vi "ChangePWMDutyCycle.vi"(4 "Duty cycle (%)":dbl=50.0, 5 "Channel":i32, 6 "error in":errorcluster) -> (0 "error out":errorcluster)   [LabVIEW 2014]
doc: "Change the duty cycle of the PWM waveform.\n\nThe channel must be configured for PWM before calling this VI."
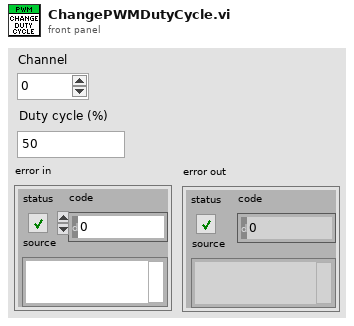
[diagram p1: front panel]
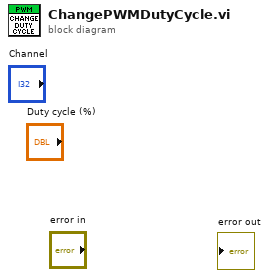
[diagram p0: block diagram]
diagram:
